vi "Import Custom Device Configuration.vi"(6 "Pre-Import Action":refnum<vi>, 7 "Overwrite Existing?":bool=TRUE, 8 "error in (no error)":errorcluster, 9 "File Interface (.dat)":refnum<class "File Interface.lvclass">=refnum, 10 "Path":path, 11 "NodeID":u64) -> (0 "error out":errorcluster, 2 "cancelled":bool, 3 "NodeID out":u64)   [LabVIEW 2019, in "ImportExport.lvlib"]
doc: "ImportCDConfig.vi loads a configuration file (.dat) previously created using ExportCDConfig.vi. This configuration file includes the values for the properties of each Section, Channel, or Waveform in your Custom Device. It is strongly recommended to call this VI from your Initialization VI."
uses:
  ImportExport.lvlib
  <vilib>/NI/NI VeriStand Custom Device Import and Export Tool/File Interface Class/File Interface.lvclass
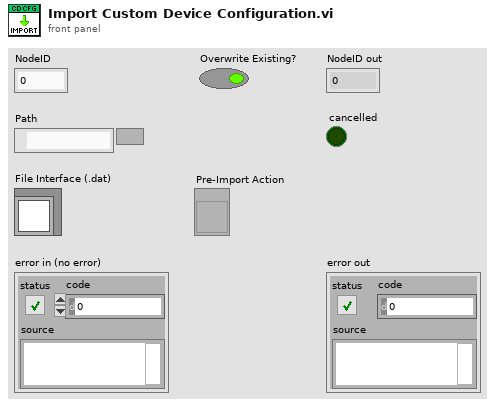
[diagram p1: front panel]
types:
  T1 = typedef "Advanced System Definition.lvlib/SysDef.Export.ctl" = cluster{"Version":string, "Tree":T2[]}
  T2 = typedef "Advanced System Definition.lvlib/TreeItem.ctl" = cluster{"Item Info":T3, "Parent Path":string[], "Properties":T8[]}
  T3 = typedef "Advanced System Definition.lvlib/TreeItem.Info.ctl" = cluster{"Name":string, "Description":string, "GUID":string, "Is Channel":bool, "Channel":T4, "Is Waveform":bool, "Waveform":T6}
  T4 = typedef "Custom Device API.lvlib/Custom Device Channel.ctl" = cluster{"Type":T5, "Units":string, "Default Value":dbl, "Faultable":bool, "Scalable":bool}
  T5 = typedef "Custom Device API.lvlib/Custom Device Channel Type.ctl" = enum16{"Input", "Output"}
  T6 = typedef "Custom Device API.lvlib/Custom Device Waveform.ctl" = cluster{"Data Type":T7, "Units":string}
  T7 = typedef "Custom Device API.lvlib/Custom Device Waveform DataType.ctl" = enum16{"Double", "Complex Double"}
  T8 = typedef "Advanced System Definition.lvlib/TreeItem.Property.ctl" = cluster{"Name":string, "Type":i32, "Value":variant}
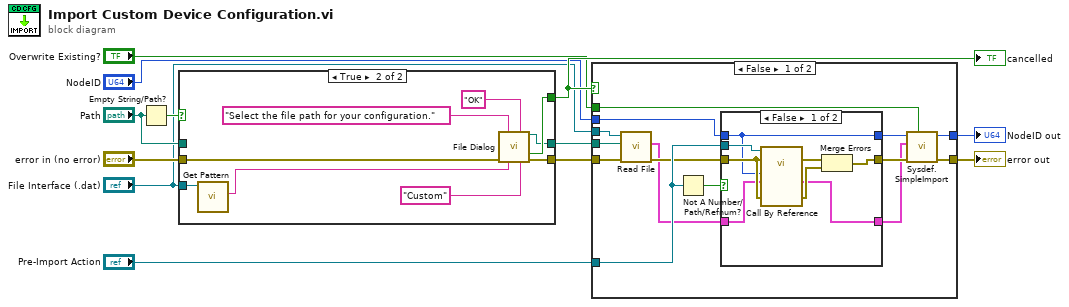
[diagram p0: block diagram]
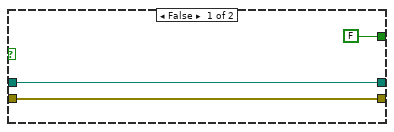
[diagram p2: hidden frame]
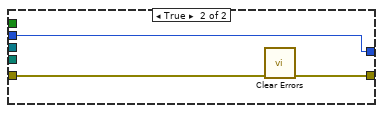
[diagram p4: hidden frame]
diagram:
  n1 = Empty String/Path?(string/path="Path") -> (empty?=w9:bool)
  n2 = case shown="True" w9 {
    tunnel: [FALSE ("cancelled") w21] -> w12
    tunnel: [w13 w20] -> w11
    tunnel: [w14 w19] -> w10
    tunnel: "error in (no error)" -> [w13 w18]
    tunnel: "Path" -> [w14 _]
    tunnel: "File Interface (.dat)" -> [_ w17]
    frame False {
    }
    frame True {
      n3 = call-dynamic "Get Pattern.vi"("File Interface in"=w17) -> ("file extension"=w16:string)  [unwired: 10 in]
      n4 = call "File Dialog"("prompt"="Select the file path for your configuration.", "button label"="OK", "error in"=w18, "pattern (all files)"=w16, "pattern label"="Custom") -> ("selected path"=w19:path, "cancelled"=w21:bool, "error out"=w20:errorcluster)  [unwired: 7 in, 1 out]
    }
  }
  "cancelled" <- w12
  n5 = case shown="False" w12 {
    tunnel: [w38 w51] -> w3
    tunnel: w11 -> [w33 w52]
    tunnel: w10 -> [w34 _]
    tunnel: "NodeID" -> [w31 w50]
    tunnel: [w37 w50] -> w5
    tunnel: "Overwrite Existing?" -> [w36 _]
    tunnel: "File Interface (.dat)" -> [w35 _]
    tunnel: "Pre-Import Action" -> [w30 _]
    frame False {
      n6 = call-dynamic "Read File.vi"("error in (no error)"=w33, "Path in"=w34, "File Interface in"=w35) -> ("error out"=w29:errorcluster, "SysDef"=w27:T1)  [unwired: 7 in]
      n7 = Not A Number/Path/Refnum?(number/path/refnum=w30) -> (NaN/Path/Refnum?=w32:bool)
      n8 = case shown="False" w32 {
        tunnel: w31 -> [w40 w48]
        tunnel: w30 -> [w46 _]
        tunnel: w29 -> [w44 w47]
        tunnel: [w43 w47] -> w28
        tunnel: w27 -> [w41 w49]
        tunnel: [w39 w49] -> w26
        tunnel: [w40 w48] -> w25
        frame False {
          n9 = call-by-ref "?"(reference=w46, error in=w44, 8:"error in (no error)"=w44, "SysDef in"=w41, "Item Ref in"=w40) -> (error out=w45:errorcluster, 0:"error out"=w42:errorcluster, "SysDef out"=w39:T1)  [unwired: 6 in, 2 out]
          n10 = Merge Errors(w45, w42) -> (w43:errorcluster)
        }
        frame True {
        }
      }
      n11 = call "Sysdef.SimpleImport.vi"("Overwrite Existing?"=w36, "error in (no error)"=w28, "SysDef"=w26, "NodeID"=w25) -> ("error out"=w38:errorcluster, "NodeID out"=w37:u64)  [unwired: 6 in]
    }
    frame True {
      n12 = call <vilib>:"Clear Errors.vi"("error in (no error)"=w52) -> ("error out"=w51:errorcluster)  [unwired: 5 in, 1 out]
    }
  }
  "error out" <- w3
  "NodeID out" <- w5
